vi "Main.vi"() -> ()   [LabVIEW 2017]
doc: "Use this template to build a simple state machine design pattern. Each state executes code and determines which state to transition to."
uses:
  controls/app_data.ctl
  controls/instruments.ctl
  Unicorn Labview Library/Control/unicorn_Param.ctl
  Unicorn Labview Library/Control/unicorn_conn.ctl
  Unicorn Labview Library/Control/unicorn_JSON.ctl
  Unicorn Labview Library/Control/unicorn_ParamInt.ctl
  Unicorn Labview Library/Control/unicorn_Telemetry.ctl
  Unicorn Labview Library/Control/unicorn_Table.ctl
  Unicorn Labview Library/Control/unicorn_ParamFloat.ctl
  controls/State.ctl
  <instrlib>/PICOTEST M352XA/Public/Controls/Function.ctl
  controls/attenuator_dB.ctl
  Unicorn Labview Library/Unicorn Library.lvlib
  <instrlib>/Siglent SDG X Series/Siglent SDG X Series.lvlib
panel:
  in  "app_data":T1={"Instruments"={"generator"="", "voltment_with_scaner"="", "voltment_without_scaner"=""}, "boc"={"conParam"={"ReadIntParam"=TRUE, "ReadDescrParam"=FALSE, "ReadFloatParam"=TRUE, "debug"=FALSE, "ReadJSON"=TRUE, "IP_address"="192.168.1.216", "N_attempts"=3, "type_con"=enum."TCP", "MB_address"=1, "VISA"="COM1", "connection ID"=refnum, "nameDevices"="", "timeout"=3000, "port"=2000, "type_version"="0F0C0001", "baud_rate"=115200, "VersionControl"=FALSE, "TCP_conn"=FALSE, "WindowSize"=700}, "Param"={"NumParam"={"NTelem"=0, "NInt"=0, "NFloat"=0, "NTable"=0}, "ParamInt"=[], "Telemetry"=[], "Table"=[], "ParamFloat"=[]}}, "boe"={"conParam"={"ReadIntParam"=TRUE, "ReadDescrParam"=FALSE, "ReadFloatParam"=TRUE, "debug"=FALSE, "ReadJSON"=TRUE, "IP_address"="192.168.1.216", "N_attempts"=3, "type_con"=enum."TCP", "MB_address"=1, "VISA"="COM1", "connection ID"=refnum, "nameDevices"="", "timeout"=3000, "port"=2000, "type_version"="0F0C0001", "baud_rate"=115200, "VersionControl"=FALSE, "TCP_conn"=FALSE, "WindowSize"=700}, "Param"={"NumParam"={"NTelem"=0, "NInt"=0, "NFloat"=0, "NTable"=0}, "ParamInt"=[], "Telemetry"=[], "Table"=[], "ParamFloat"=[]}}, "attenuator_tune_koef"=[]}
  out "voltmetr 3":bool
  in  "voltmetr_wothout_scaner":refnum<visa-resource-name>="voltmetr_without_scanner" caption="Вольтметр без сканера (перед аттенюатором)"
  in  "Exit":bool
  out "error out 2":errorcluster
  out "boe_connected":bool caption="Соединение"
  in  "Connect_boe":bool caption="Подключение"
  out "voltmetr":bool
  out "generator":bool
  in  "voltmetr_with_scaner":refnum<visa-resource-name>="USB0::0x164E::0x0DAD::TW00054344::INSTR" caption="Вольтметр со сканером"
  in  "generator":refnum<visa-resource-name>="generator" caption="Генератор"
  out "boc_connected":bool caption="Соединение"
  in  "Tab Control":T10(tab)
  in  "frequencies":dbl[](array[numeric])=[50000.0, 60000.0, 70000.0, 80000.0, 90000.0, 100000.0, 110000.0, 120000.0, 130000.0, 140000.0, 150000.0, 160000.0, 170000.0, 180000.0, 190000.0, 200000.0, 210000.0, 220000.0, 230000.0, 240000.0, 250000.0] format="%#_6p"
  in  "attenuator_setup":bool
  out "appended array":dbl[][](array[numeric]) format="%#_6p"
  out "после аттенюатора":dbl[](array[numeric])
  out "error out 7":errorcluster
  in  "icp_check":bool
  out "error out 3":errorcluster
  out "Telemetry 2":sgl[][](array[numeric])
  in  "calibration":bool
  out "error out 4":errorcluster
  out "meas":dbl[](array[numeric])
  out "boc_data":sgl[](array[numeric])
  out "koef":dbl[](array[numeric])
  out "meas 2":dbl[](array[numeric])
  out "boc_data 2":sgl[](array[numeric])
  out "koef 2":dbl[](array[numeric])
  in  "check_calibr":bool
  out "meas 3":dbl[](array[numeric])
  out "boc_data 3":sgl[](array[numeric])
  out "koef 3":dbl[](array[numeric])
  out "meas 4":dbl[](array[numeric])
  out "boc_data 4":sgl[](array[numeric])
  out "koef 4":dbl[](array[numeric])
  out "error out 5":errorcluster
  in  "meas_freq_char":bool
  in  "freq":dbl[](array[numeric])=[50000.0, 60000.0, 70000.0, 100000.0, 140000.0, 180000.0, 210000.0, 250000.0] caption="Частоты" format="%#_6p"
  out "error out 6":errorcluster
  in  "Tab Control 2":T11(tab)
  out "meas 5":dbl[][](array[numeric])
  out "boc_data 5":sgl[][](array[numeric])
  out "meas 6":dbl[][](array[numeric])
  out "boc_data 6":sgl[][](array[numeric])
  out "boc_data 10":sgl[][](array[numeric])
  out "meas 9":dbl[][](array[numeric])
  in  "voltage":dbl[](array[numeric])=[0.0001, 0.0005, 0.001, 0.005, 0.01, 0.05, 0.1, 0.14] min=0.0 max=1.0 format="%#_6p"
  in  "ampl_char_without_atten":bool
  out "error out 8":errorcluster
  in  "Tab Control 3":T11(tab)
  out "meas 7":dbl[][](array[numeric])
  out "boc_data 7":sgl[][](array[numeric])
  out "meas 8":dbl[][](array[numeric])
  out "boc_data 8":sgl[][](array[numeric])
  out "meas 10":dbl[][](array[numeric])
  out "boc_data 11":sgl[][](array[numeric])
  in  "cross_channel_links":bool
  out "boc_data 9":sgl[][](array[numeric])
  out "error out 9":errorcluster
  in  "Connect_boc":bool caption="Подключение"
  out "error out":errorcluster
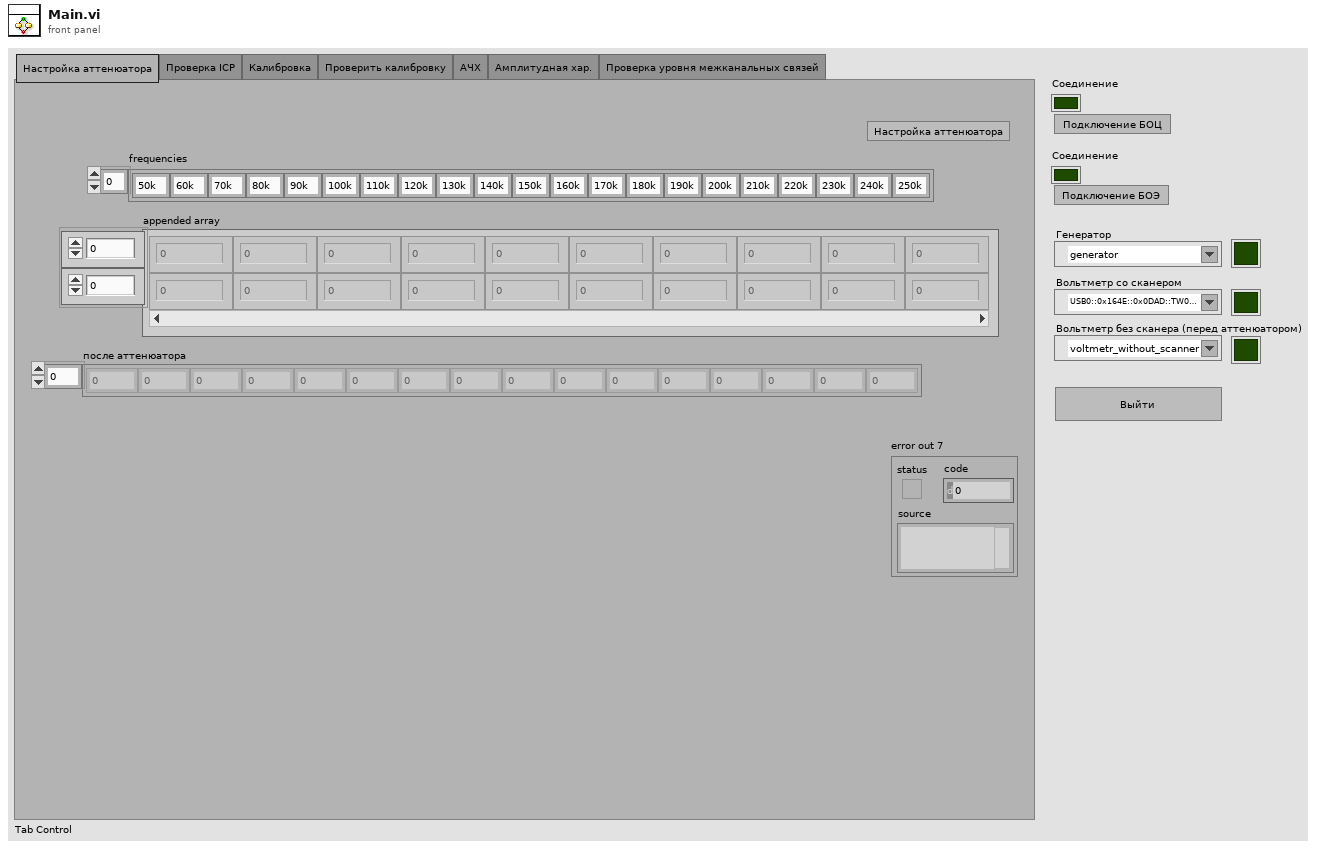
[diagram p1: front panel]
types:
  T1 = typedef "app_data.ctl" = cluster{"Instruments":T2, "boc":T3, "boe":T3, "attenuator_tune_koef":dbl[][]}
  T2 = typedef "instruments.ctl" = cluster{"generator":refnum<visa-resource-name>, "voltment_with_scaner":refnum<visa-resource-name>, "voltment_without_scaner":refnum<visa-resource-name>}
  T3 = typedef "Unicorn Library.lvlib/unicorn_Param.ctl" = cluster{"conParam":T4, "Param":T5}
  T4 = typedef "Unicorn Library.lvlib/unicorn_conn.ctl" = cluster{"ReadIntParam":bool, "ReadDescrParam":bool, "ReadFloatParam":bool, "debug":bool, "ReadJSON":bool, "IP_address":string, "N_attempts":i32, "type_con":enum16{"Serial", "TCP"}, "MB_address":i32, "VISA":refnum<visa-resource-name>, "connection ID":refnum<k5>, "nameDevices":string, "timeout":i32, "port":u16, "type_version":string, "baud_rate":u32, "VersionControl":bool, "TCP_conn":bool, "WindowSize":i32}
  T5 = typedef "Unicorn Library.lvlib/unicorn_JSON.ctl" = cluster{"NumParam":cluster{"NTelem":i32, "NInt":i32, "NFloat":i32, "NTable":i32}, "ParamInt":T6, "Telemetry":T7, "Table":T8, "ParamFloat":T9}
  T6 = typedef "Unicorn Library.lvlib/unicorn_ParamInt.ctl" = cluster{"ID":string, "Num":i32, "Name":string, "Type":string, "Enum":string, "Desc":string, "Unit":string, "Access":string, "FormatStr":string, "Min":i32, "Max":i32}[]
  T7 = typedef "Unicorn Library.lvlib/unicorn_Telemetry.ctl" = cluster{"ID":string, "Num":i32, "Name":string, "Desc":string, "Unit":string, "FormatStr":string, "Min":i32, "Max":i32}[]
  T8 = typedef "Unicorn Library.lvlib/unicorn_Table.ctl" = cluster{"Num":i32, "Access":string, "ColumnCount":i32, "NeedParamPrepare":bool, "Columns":cluster{"Column":i32, "Desc":string, "Name":string}[], "DataType":string, "FormatStr":string, "ID":string, "Name":string, "RowCount":i32, "Rows":cluster{"Desc":string, "ID":string, "Max":i32, "Min":i32, "Name":string, "Row":i32, "Unit":string}[], "Type":string}[]
  T9 = typedef "Unicorn Library.lvlib/unicorn_ParamFloat.ctl" = cluster{"ID":string, "Num":i32, "Name":string, "Type":string, "Enum":string, "Desc":string, "Unit":string, "Access":string, "FormatStr":string, "Min":i32, "Max":i32}[]
  T10 = enum32{"Настройка аттенюатора", "Проверка ICP", "Калибровка", "Проверить калибровку", "АЧХ", "Амплитудная хар.", "Проверка уровня межканальных связей"}
  T11 = enum32{"BOE -1, BOC 0", "BOE -1, BOC 3", "BOE 0, BOC 0"}
  T12 = typedef "State.ctl" = enum16{"Initialize", "Wait for Event", "User State 1", "User State 2", "Exit"}
  T13 = typedef "Function.ctl" = enum16{"VOLTage:DC", "VOLTage:DC:RATio", "VOLTage:AC", "CURRent:DC", "CURRent:AC", "RESistance", "FRESistance", "FREQuency", "PERiod", "FREQuency:CURRent", "PERiod:CURRent", "CAPacitance", "CONTinuity", "DIODe", "TCOuple", "TEMPerature"}
  T14 = typedef "attenuator_dB.ctl" = enum16{"0", "20", "40", "60"}
  T15 = typedef "Unicorn Library.lvlib/AnswerUDP.ctl" = cluster{"IP":string, "Port":u16, "DataVersion":u16, "ModbusAddress":i32, "type_version":string, "Description":string, "Serial":string, "ServerPort":u16}
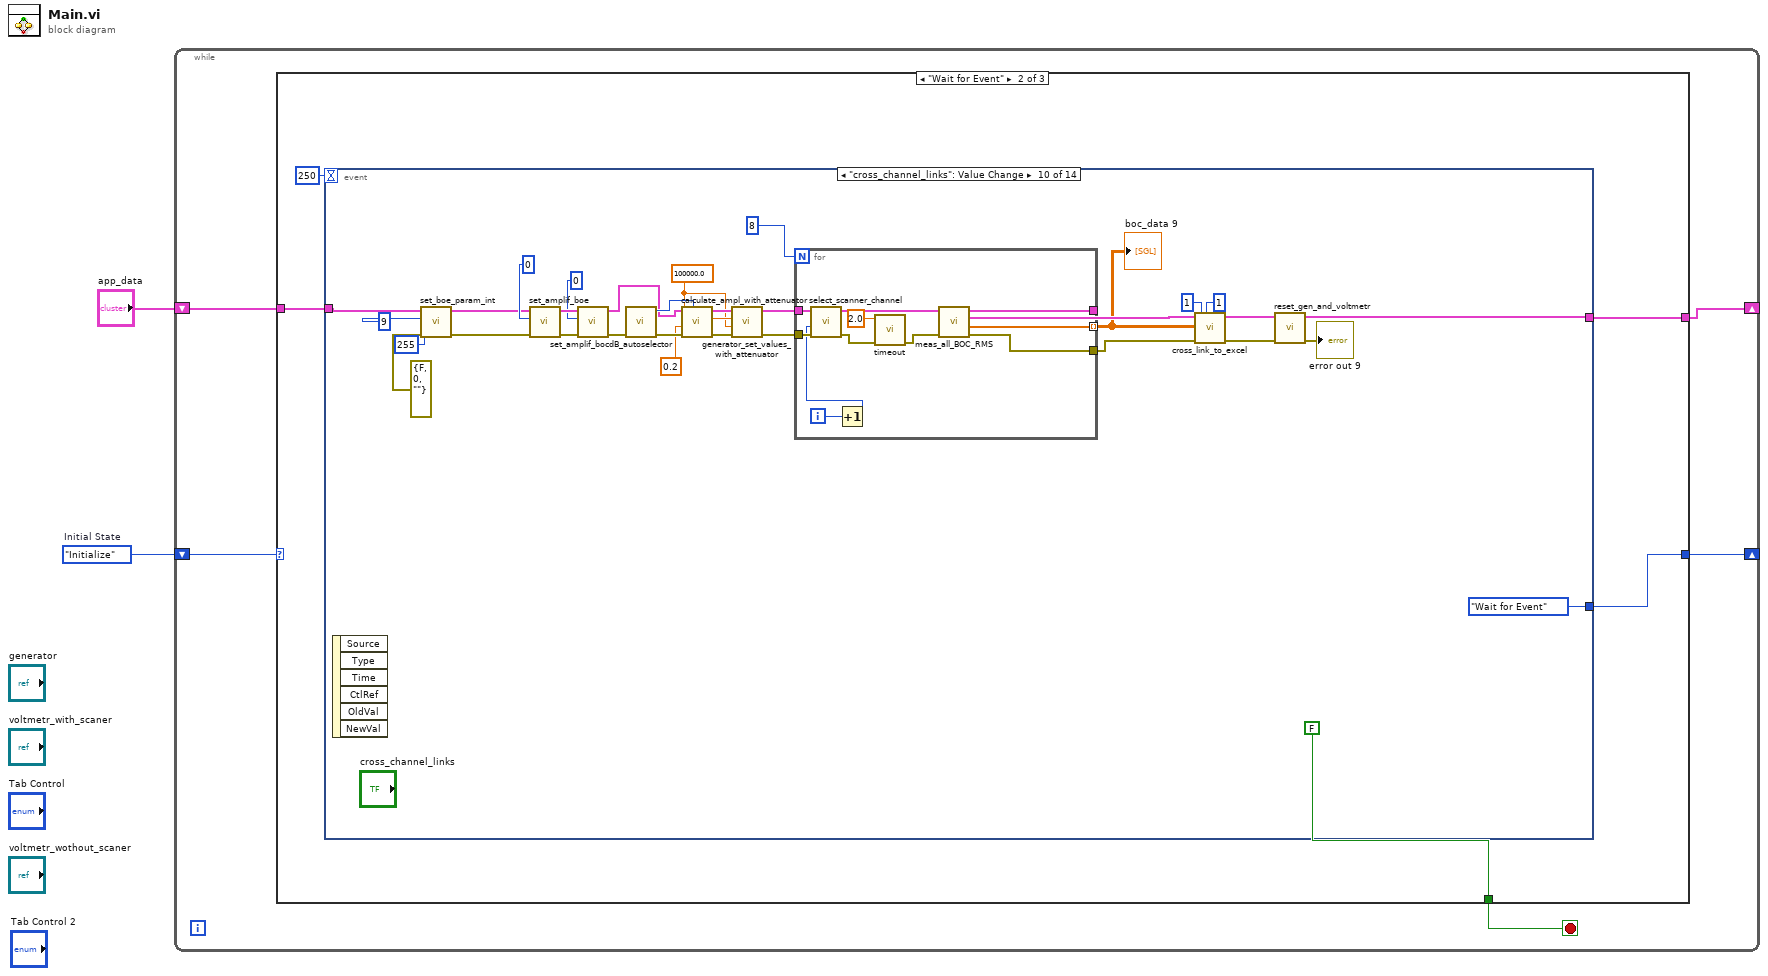
[diagram p0: block diagram]
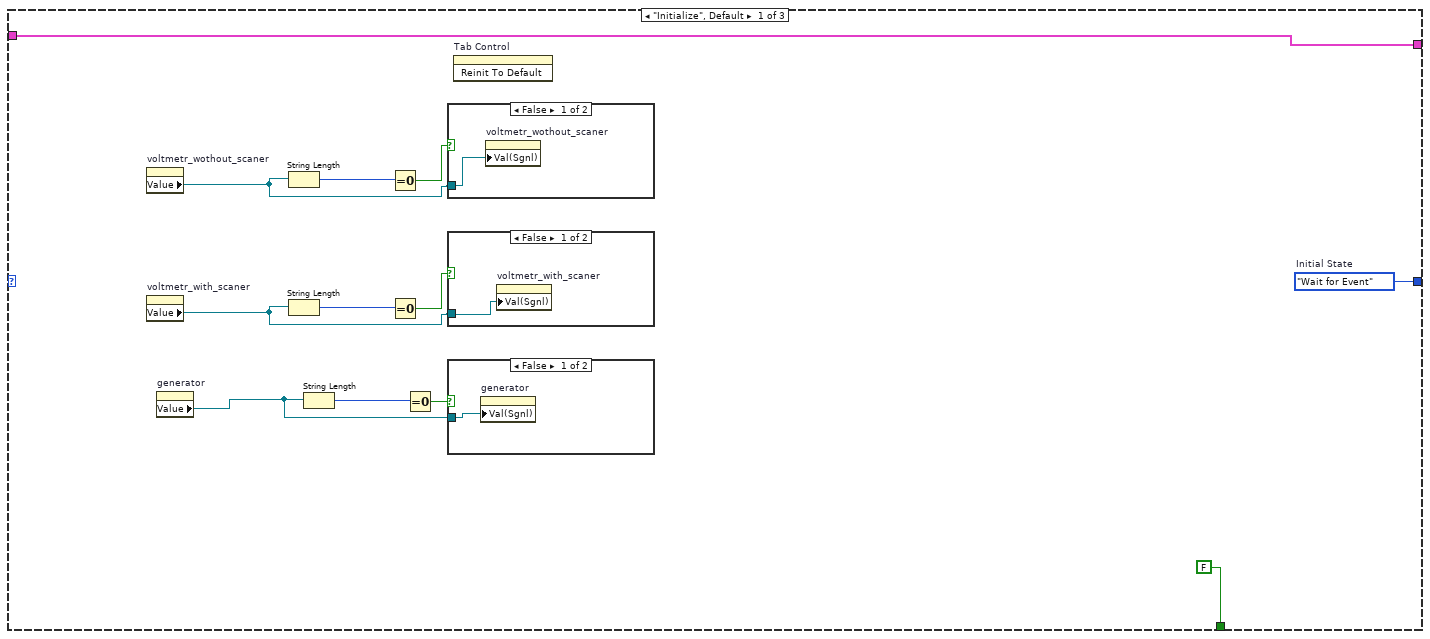
[diagram p2: hidden frame]
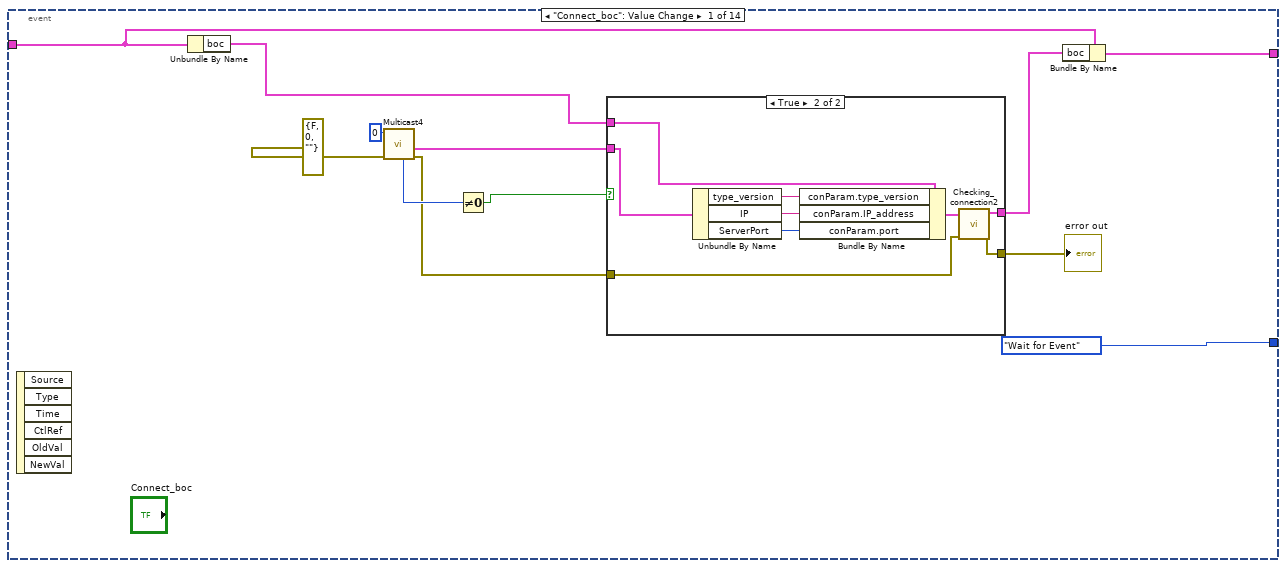
[diagram p6: hidden frame]
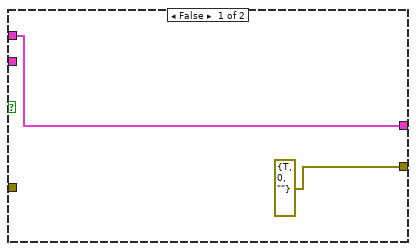
[diagram p7: hidden frame]
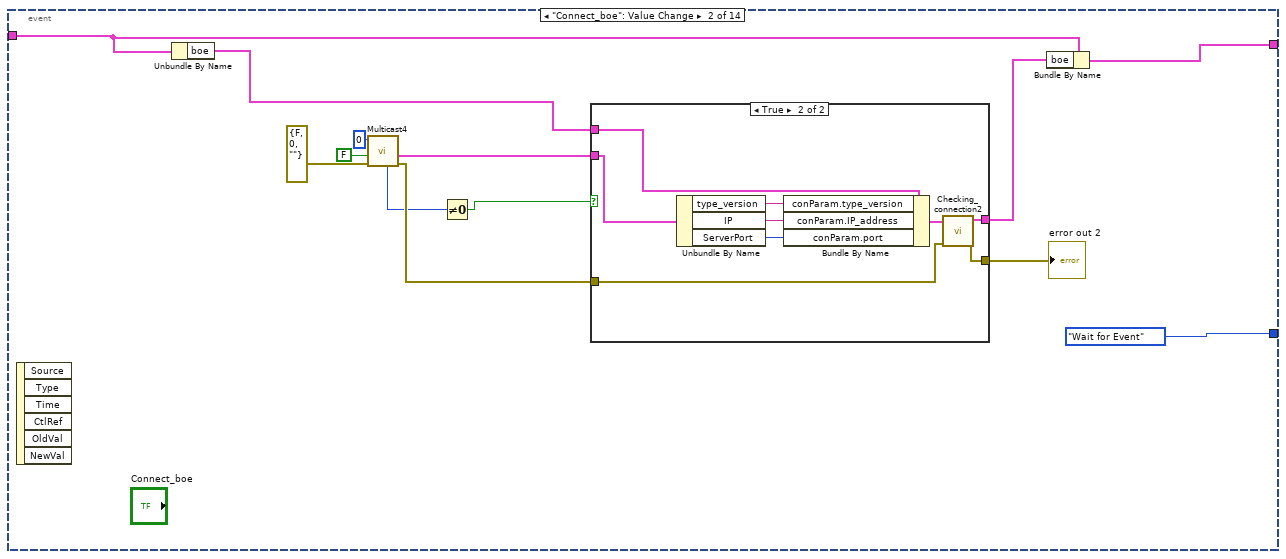
[diagram p8: hidden frame]
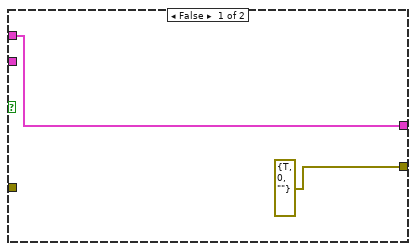
[diagram p9: hidden frame]
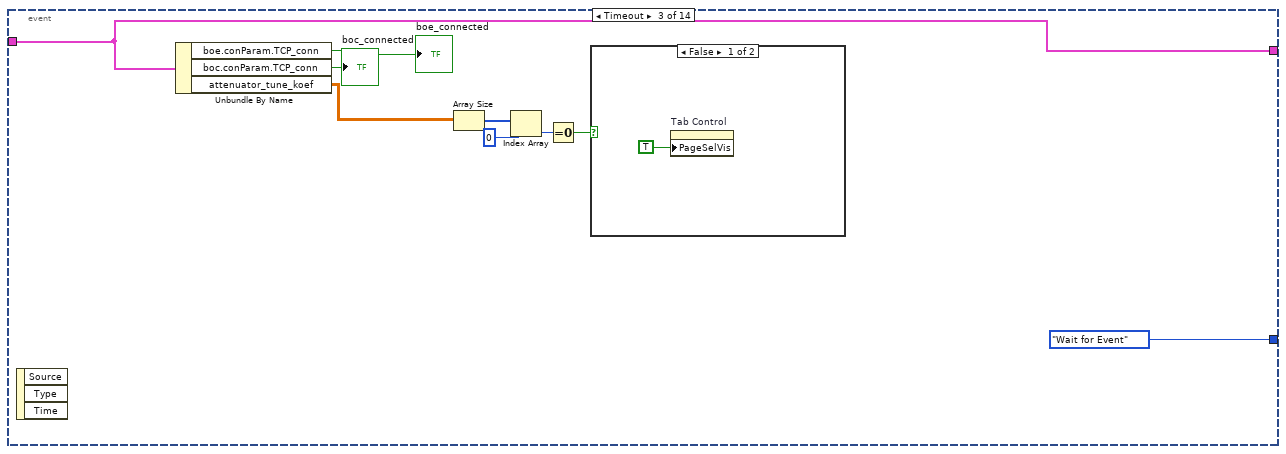
[diagram p10: hidden frame]
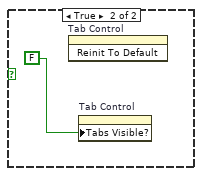
[diagram p11: hidden frame]
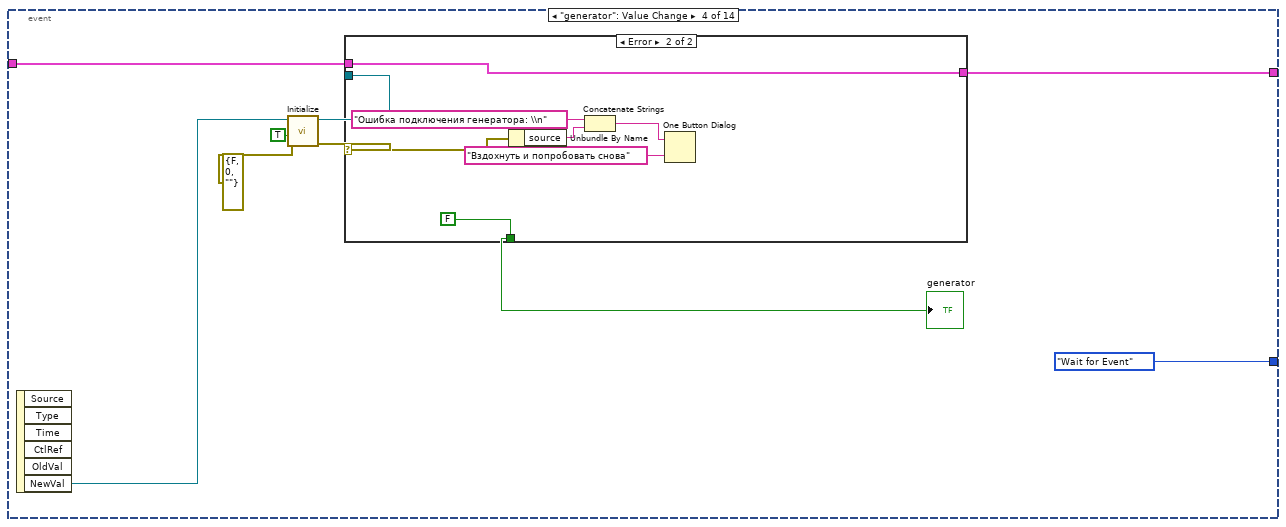
[diagram p12: hidden frame]
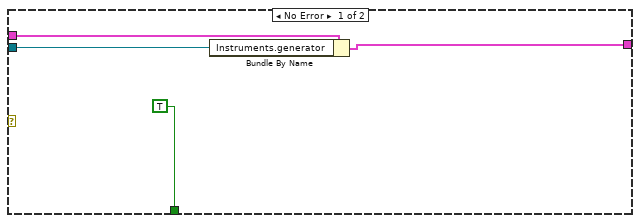
[diagram p13: hidden frame]
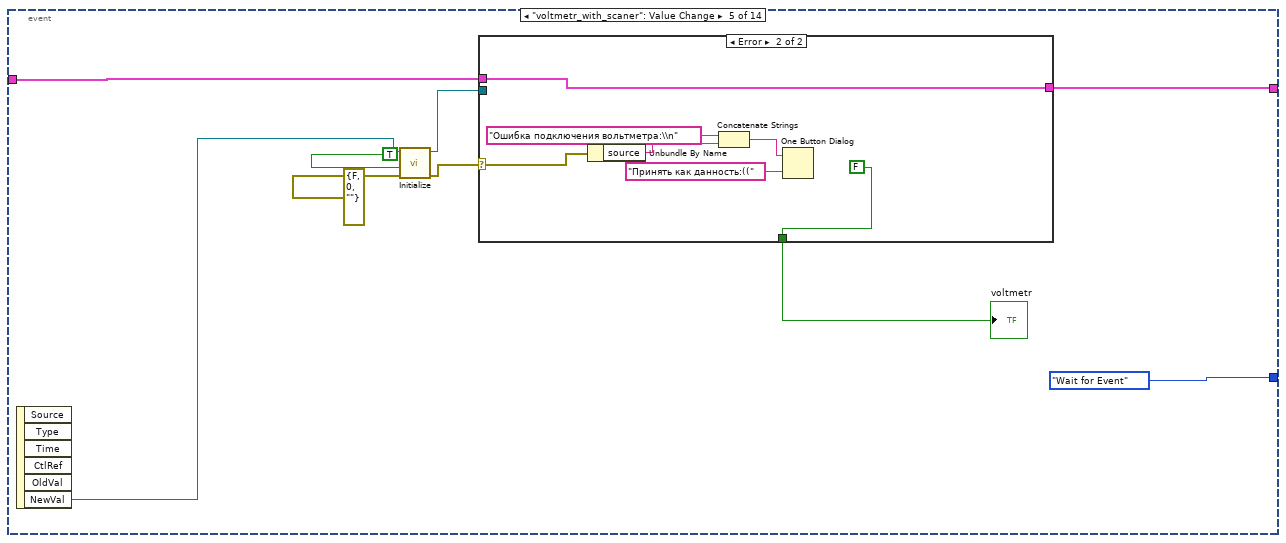
[diagram p14: hidden frame]
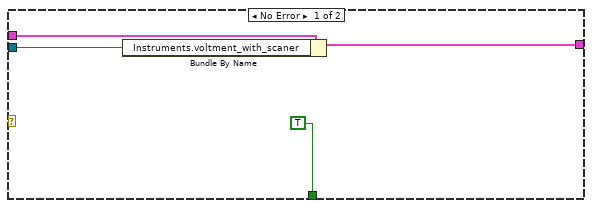
[diagram p15: hidden frame]
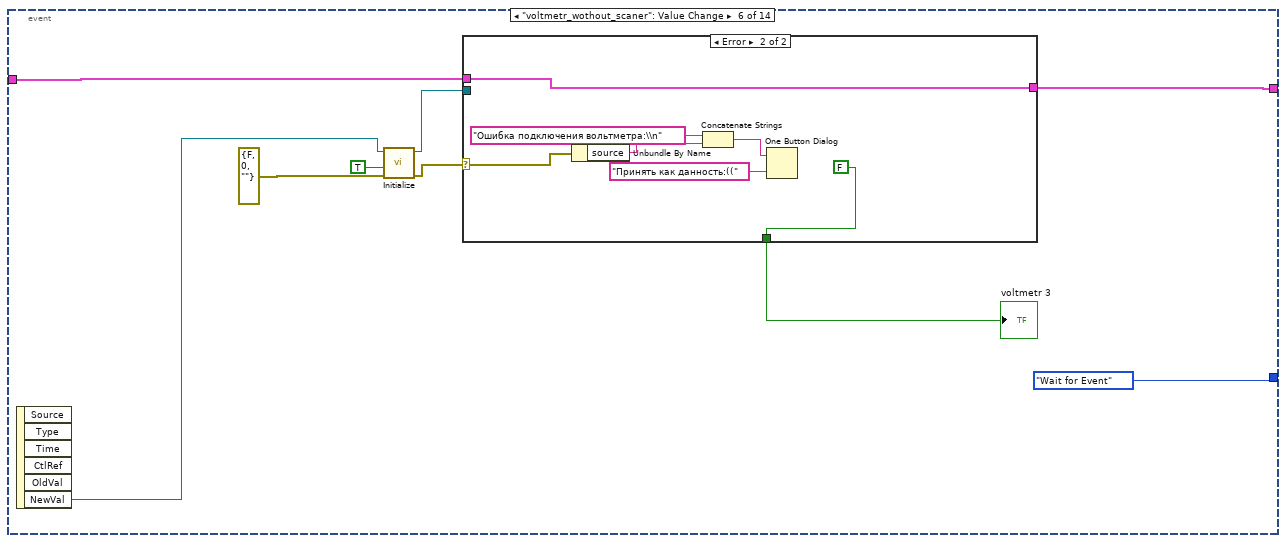
[diagram p16: hidden frame]
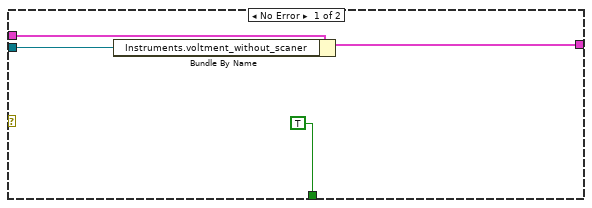
[diagram p17: hidden frame]
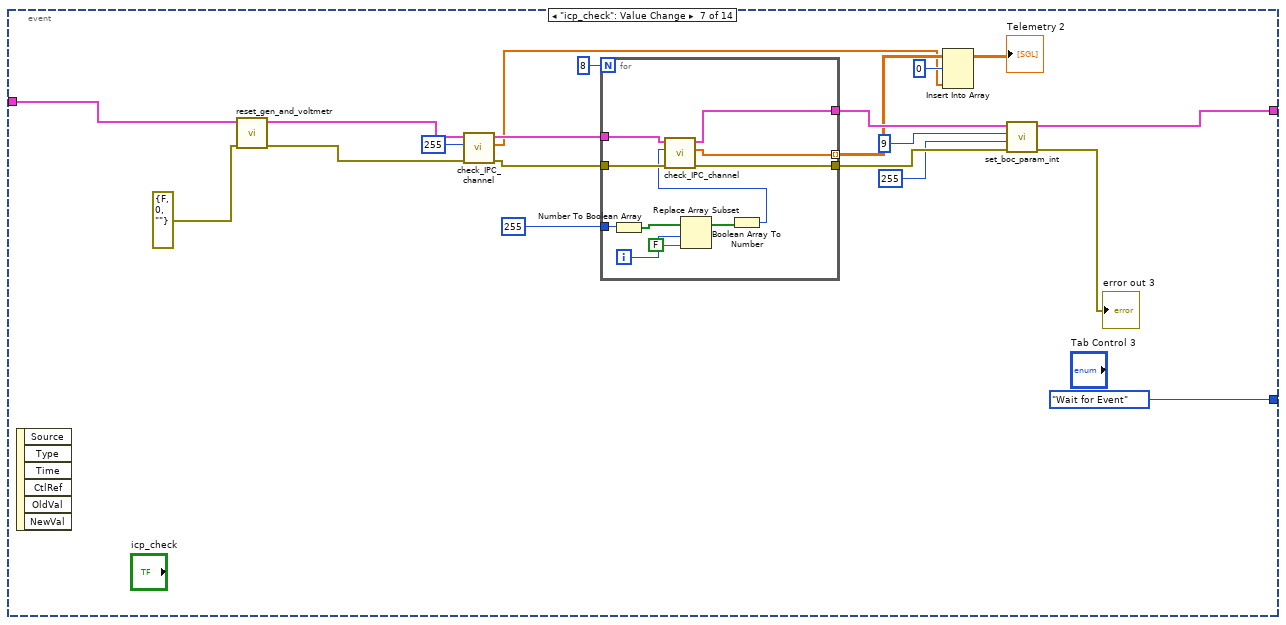
[diagram p18: hidden frame]
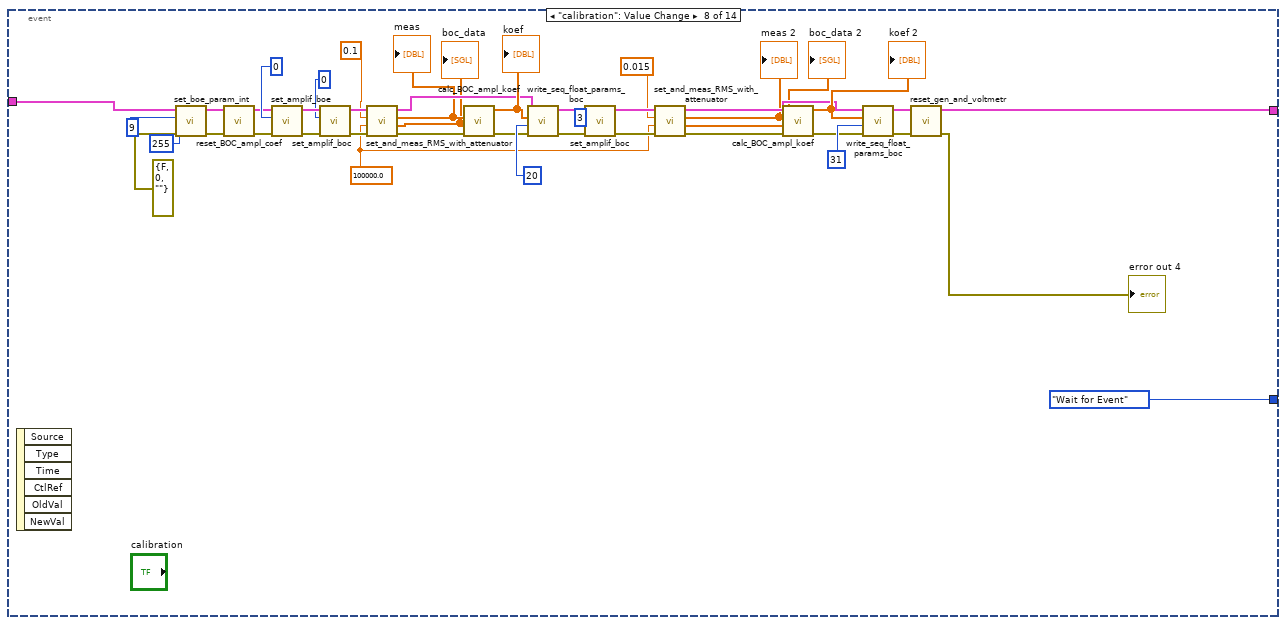
[diagram p19: hidden frame]
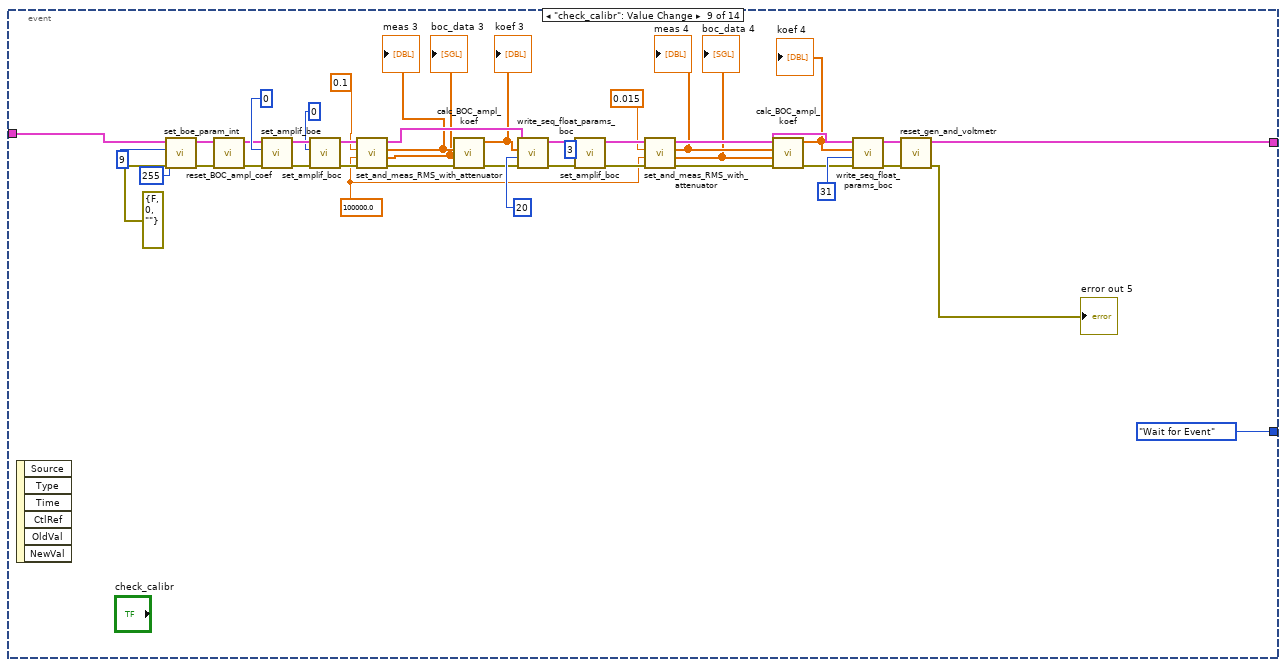
[diagram p20: hidden frame]
diagram:
  w2 = State."Initialize"  # Initial State
  n1 = while {
    shift-right: [w3] -> _
    shift-left: w2 -> [w7]
    shift-right: [w4] -> _
    shift-left: "app_data" -> [w6]
    stop <- w5 stop-if-true
    n2 = case shown="\"Wait for Event\"" w7 {
      tunnel: [w17 w25 w473] -> w4
      tunnel: w6 -> [w17 w26 w473]
      tunnel: [w19 w24 w472] -> w3
      tunnel: [FALSE FALSE TRUE] -> w5
      frame "Initialize", Default {
        w19 = State."Wait for Event"  # Initial State
        n3 = property on="voltmetr_wothout_scaner" class="VISAName"() -> ("Value"=w8:refnum<visa-resource-name>)  [unwired: 2 in, 2 out]
        n4 = property on="voltmetr_with_scaner" class="VISAName"() -> ("Value"=w11:refnum<visa-resource-name>)  [unwired: 2 in, 2 out]
        n5 = property on="generator" class="VISAName"() -> ("Value"=w14:refnum<visa-resource-name>)  [unwired: 2 in, 2 out]
        n6 = String Length(string=w8) -> (length=w9:i32)
        n7 = String Length(string=w11) -> (length=w13:i32)
        n8 = String Length(string=w14) -> (length=w16:i32)
        n9 = Equal To 0?(x=w9) -> (x = 0?=w10:bool)
        n10 = Equal To 0?(x=w13) -> (x = 0?=w12:bool)
        n11 = Equal To 0?(x=w16) -> (x = 0?=w15:bool)
        n12 = case shown="False" w10 {
          tunnel: w8 -> [w20 _]
          frame False {
            n13 = property on="voltmetr_wothout_scaner" class="VISAName"("Val(Sgnl)"=w20) -> ()  [unwired: 2 in, 2 out]
          }
          frame True {
          }
        }
        n14 = case shown="False" w12 {
          tunnel: w11 -> [w21 _]
          frame False {
            n15 = property on="voltmetr_with_scaner" class="VISAName"("Val(Sgnl)"=w21) -> ()  [unwired: 2 in, 2 out]
          }
          frame True {
          }
        }
        n16 = case shown="False" w15 {
          tunnel: w14 -> [w22 _]
          frame False {
            n17 = property on="generator" class="VISAName"("Val(Sgnl)"=w22) -> ()  [unwired: 2 in, 2 out]
          }
          frame True {
          }
        }
        n18 = invoke on="Tab Control" class="TabCtl (strict)" method="Reinit To Default"() -> ()  [unwired: 3 in, 3 out]
      }
      frame "Wait for Event" {
        n19 = event shown="[9] \"cross_channel_links\": Value Change" {
          selector: _ -> [_ _ _ _ _ _ _ _ _ _ _ _ _ _]
          dyn-events: _ -> [_ _ _ _ _ _ _ _ _ _ _ _ _ _]
          timeout: 250 -> [_ _ _ _ _ _ _ _ _ _ _ _ _ _]
          tunnel: w26 -> [w38 w53 w82 w91 w114 w130 w162 w217 w224 w283 w323 w384 w407 w464]
          tunnel: [w39 w54 w82 w89 w113 w129 w153 w194 w225 w268 w316 w383 w408 w464] -> w25
          tunnel: [State."Wait for Event" ("Initial State") State."Wait for Event" ("Initial State") State."Wait for Event" ("Initial State") State."Wait for Event" ("Initial State") State."Wait for Event" ("Initial State") State."Wait for Event" ("Initial State") State."Wait for Event" ("Initial State") State."Wait for Event" ("Initial State") State."Wait for Event" ("Initial State") State."Wait for Event" ("Initial State") State."Wait for Event" ("Initial State") State."Wait for Event" ("Initial State") State."Wait for Event" ("Initial State") State."Exit" ("Initial State")] -> w24
          event "Connect_boc": Value Change {
            n20 = event-data() -> ()  [unwired: 1 in, 6 out]
            n21 = Unbundle By Name(w38) -> ("boc"=w31:T3)
            n22 = call "Multicast4.vi"("error in"=errorcluster {"status"=FALSE, "code"=0, "source"=""} ("error in (no error)"), "type_version"=u32 0) -> ("error out"=w29:errorcluster, "selDevice"=w32:T15, "selIPhex"=w35:u32)  [unwired: 4 in, 3 out]
            n23 = Not Equal To 0?(x=w35) -> (x != 0?=w34:bool)
            n24 = case shown="True" w34 {
              tunnel: [errorcluster {"status"=TRUE, "code"=0, "source"=""} ("error out") w45] -> w33
              tunnel: w32 -> [_ w47]
              tunnel: w31 -> [w40 w46]
              tunnel: [w40 w43] -> w30
              tunnel: w29 -> [_ w42]
              frame False {
              }
              frame True {
                n25 = Unbundle By Name(w47) -> ("type_version"=w49:string, "IP"=w50:string, "ServerPort"=w48:u16)
                n26 = Bundle By Name(cluster=w46, "conParam.type_version"=w49, "conParam.IP_address"=w50, "conParam.port"=w48) -> (w44:T3)
                n27 = call "Checking_connection2.vi"("error in"=w42, "paramUnicornIn"=w44) -> ("error out"=w45:errorcluster, "paramUnicorn"=w43:T3)  [unwired: 6 in, 2 out]
              }
            }
            "error out" <- w33
            n28 = Bundle By Name(cluster=w38, "boc"=w30) -> (w39:T1)
          }
          event "Connect_boe": Value Change {
            n29 = event-data() -> ()  [unwired: 1 in, 6 out]
            n30 = Unbundle By Name(w53) -> ("boe"=w61:T3)
            n31 = call "Multicast4.vi"("error in"=errorcluster {"status"=FALSE, "code"=0, "source"=""} ("error in (no error)"), "VersionControl"=FALSE, "type_version"=u32 0) -> ("error out"=w63:errorcluster, "selDevice"=w60:T15, "selIPhex"=w57:u32)  [unwired: 3 in, 3 out]
            n32 = Not Equal To 0?(x=w57) -> (x != 0?=w58:bool)
            n33 = case shown="True" w58 {
              tunnel: [errorcluster {"status"=TRUE, "code"=0, "source"=""} ("error out") w69] -> w59
              tunnel: w60 -> [_ w71]
              tunnel: w61 -> [w64 w70]
              tunnel: [w64 w67] -> w62
              tunnel: w63 -> [_ w66]
              frame False {
              }
              frame True {
                n34 = Unbundle By Name(w71) -> ("type_version"=w73:string, "IP"=w74:string, "ServerPort"=w72:u16)
                n35 = Bundle By Name(cluster=w70, "conParam.type_version"=w73, "conParam.IP_address"=w74, "conParam.port"=w72) -> (w68:T3)
                n36 = call "Checking_connection2.vi"("error in"=w66, "paramUnicornIn"=w68) -> ("error out"=w69:errorcluster, "paramUnicorn"=w67:T3)  [unwired: 6 in, 2 out]
              }
            }
            "error out 2" <- w59
            n37 = Bundle By Name(cluster=w53, "boe"=w62) -> (w54:T1)
          }
          event Timeout {
            n38 = event-data() -> ()  [unwired: 1 in, 3 out]
            n39 = Unbundle By Name(w82) -> ("boe.conParam.TCP_conn"=→"boe_connected":bool, "boc.conParam.TCP_conn"=→"boc_connected":bool, "attenuator_tune_koef"=w79:dbl[][])
            n40 = Array Size(array=w79) -> (size(s)=w78:i32[])
            n41 = Index Array(array=w78, index=0) -> (element=w76:i32)
            n42 = Equal To 0?(x=w76) -> (x = 0?=w75:bool)
            n43 = case shown="False" w75 {
              frame False {
                n44 = property on="Tab Control" class="TabCtl (strict)"("PageSelVis"=TRUE ("Page Selector Visible")) -> ()  [unwired: 2 in, 2 out]
              }
              frame True {
                n45 = invoke on="Tab Control" class="TabCtl (strict)" method="Reinit To Default"() -> ()  [unwired: 3 in, 3 out]
                n46 = property on="Tab Control" class="TabCtl (strict)"("Tabs Visible?"=FALSE ("Page Selector Visible")) -> ()  [unwired: 2 in, 2 out]
              }
            }
          }
          event "generator": Value Change {
            n47 = event-data() -> ("NewVal"=w88:refnum<visa-resource-name>)  [unwired: 1 in, 5 out]
            n48 = call <instrlib>:"Initialize.vi"("error in (no error)"=errorcluster {"status"=FALSE, "code"=0, "source"=""}, "Reset (True)"=TRUE, "VISA resource name"=w88) -> ("error out"=w92:errorcluster, "VISA resource name out"=w90:refnum<visa-resource-name>)  [unwired: 7 in]
            n49 = case shown="Error" w92 {
              selector: w92 -> [_ w104]
              tunnel: w91 -> [w98 w105]
              tunnel: w90 -> [w97 _]
              tunnel: [w96 w105] -> w89
              tunnel: [TRUE ("generator") FALSE ("generator")] -> w87
              frame No Error {
                n50 = Bundle By Name(cluster=w98, "Instruments.generator"=w97) -> (w96:T1)
              }
              frame Error {
                n51 = Unbundle By Name(w104) -> ("source"=w103:string)
                n52 = Concatenate Strings("Ошибка подключения генератора: \\n" ("string"), w103) -> (w102:string)
                n53 = One Button Dialog(message=w102, button name ("OK")="Вздохнуть и попробовать снова") -> ()  [unwired: 1 out]
              }
            }
            "generator" <- w87
          }
          event "voltmetr_with_scaner": Value Change {
            n54 = event-data() -> ("NewVal"=w108:refnum<visa-resource-name>)  [unwired: 1 in, 5 out]
            n55 = call <instrlib>:"Initialize.vi"("error in (no error)"=errorcluster {"status"=FALSE, "code"=0, "source"=""}, "Reset (True)"=TRUE, "VISA resource name"=w108) -> ("error out"=w110:errorcluster, "VISA resource name out"=w109:refnum<visa-resource-name>)  [unwired: 6 in, 1 out]
            n56 = case shown="Error" w110 {
              selector: w110 -> [_ w124]
              tunnel: w114 -> [w118 w125]
              tunnel: [w117 w125] -> w113
              tunnel: w109 -> [w116 _]
              tunnel: [TRUE ("voltmetr") FALSE ("voltmetr")] -> w107
              frame No Error {
                n57 = Bundle By Name(cluster=w118, "Instruments.voltment_with_scaner"=w116) -> (w117:T1)
              }
              frame Error {
                n58 = Unbundle By Name(w124) -> ("source"=w123:string)
                n59 = Concatenate Strings("Ошибка подключения вольтметра:\\n" ("string"), w123) -> (w121:string)
                n60 = One Button Dialog(message=w121, button name ("OK")="Принять как данность:((") -> ()  [unwired: 1 out]
              }
            }
            "voltmetr" <- w107
          }
          event "voltmetr_wothout_scaner": Value Change {
            n61 = event-data() -> ("NewVal"=w127:refnum<visa-resource-name>)  [unwired: 1 in, 5 out]
            n62 = call <instrlib>:"Initialize.vi"("error in (no error)"=errorcluster {"status"=FALSE, "code"=0, "source"=""}, "Reset (True)"=TRUE, "VISA resource name"=w127) -> ("error out"=w132:errorcluster, "VISA resource name out"=w131:refnum<visa-resource-name>)  [unwired: 6 in, 1 out]
            n63 = case shown="Error" w132 {
              selector: w132 -> [_ w144]
              tunnel: w130 -> [w138 w145]
              tunnel: [w137 w145] -> w129
              tunnel: w131 -> [w136 _]
              tunnel: [TRUE ("voltmetr") FALSE ("voltmetr")] -> w126
              frame No Error {
                n64 = Bundle By Name(cluster=w138, "Instruments.voltment_without_scaner"=w136) -> (w137:T1)
              }
              frame Error {
                n65 = Unbundle By Name(w144) -> ("source"=w143:string)
                n66 = Concatenate Strings("Ошибка подключения вольтметра:\\n" ("string"), w143) -> (w141:string)
                n67 = One Button Dialog(message=w141, button name ("OK")="Принять как данность:((") -> ()  [unwired: 1 out]
              }
            }
            "voltmetr 3" <- w126
          }
          event "icp_check": Value Change {
            n68 = event-data() -> ()  [unwired: 1 in, 6 out]
            n69 = call "reset_gen_and_voltmetr.vi"("error in (no error)"=errorcluster {"status"=FALSE, "code"=0, "source"=""}, "app_data"=w162) -> ("error out"=w163:errorcluster, "output cluster"=w150:T1)  [unwired: 8 in]
            n70 = call "check_IPC_channel.vi"("error in (no error)"=w163, "ParamIn"=255, "app_data in"=w150) -> ("error out"=w160:errorcluster, "Telemetry"=w147:sgl[], "app_data out"=w161:T1)  [unwired: 6 in]
            n71 = for {
              N: 8 -> [_]
              tunnel: [w176] -> w149 mode=indexing
              tunnel: w161 -> [w175]
              tunnel: [w174] -> w154
              tunnel: w160 -> [w173]
              tunnel: [w172] -> w156
              tunnel: u8 255 ("ParamIn") -> [w171]
              i -> [w169]
              n72 = Number To Boolean Array(number=w171) -> (Boolean array=w170:bool[])
              n73 = Replace Array Subset(array=w170, new element=FALSE ("new element/subarray"), index=w169) -> (w167:bool[])
              n74 = Boolean Array To Number(Boolean array=w167) -> (number=w166:u32)
              n75 = call "check_IPC_channel.vi"("error in (no error)"=w173, "ParamIn"=w166, "app_data in"=w175) -> ("error out"=w172:errorcluster, "Telemetry"=w176:sgl[], "app_data out"=w174:T1)  [unwired: 6 in]
            }
            n76 = Insert Into Array(array=w149, index (row)=0, new element=w147) -> (→"Telemetry 2":sgl[][])  [unwired: 1 in]
            n77 = call "set_boс_param_int.vi"("error in (no error)"=w156, "ParamIn"=255, "NumParamIn"=9, "app_data in"=w154) -> ("error out"=→"error out 3":errorcluster, "app_data out"=w153:T1)  [unwired: 6 in]
          }
          event "calibration": Value Change {
            w182 = 100000.0 ("Frequency (1000 Hz)")
            n78 = event-data() -> ()  [unwired: 1 in, 6 out]
            n79 = call "set_boe_param_int.vi"("error in (no error)"=errorcluster {"status"=FALSE, "code"=0, "source"=""}, "ParamIn"=255, "NumParamIn"=9, "app_data in"=w217) -> ("error out"=w205:errorcluster, "app_data out"=w206:T1)  [unwired: 6 in]
            n80 = call "reset_BOC_ampl_coef.vi"("error in (no error)"=w205, "app_data in"=w206) -> ("error out"=w207:errorcluster, "app_data_out"=w208:T1)  [unwired: 8 in]
            n81 = call "set_amplif_boe.vi"("error in (no error)"=w207, "ParamIn"=0, "app_data in"=w208) -> ("error out"=w210:errorcluster, "app_data out"=w212:T1)  [unwired: 7 in]
            n82 = call "set_amplif_boc.vi"("error in (no error)"=w210, "ParamIn"=0, "app_data in"=w212) -> ("error out"=w190:errorcluster, "app_data out"=w191:T1)  [unwired: 7 in]
            n83 = call "set_and_meas_RMS_with_attenuator.vi"("error in (no error)"=w190, "Frequency (Hz)"=w182, "Amplitude (1.0 Vpp)"=0.1, "app_data in"=w191) -> ("error out"=w185:errorcluster, "boc_data"=w186:sgl[], "meas"=w187:dbl[], "output cluster out"=w188:T1)  [unwired: 4 in]
            "meas" <- w187
            "boc_data" <- w186
            n84 = call "calc_BOC_ampl_koef.vi"("error_in"=w185, "boc_data"=w186, "meas"=w187) -> ("error_out"=w192:errorcluster, "koef"=w204:dbl[])  [unwired: 7 in]
            "koef" <- w204
            n85 = call "write_seq_float_params_boc.vi"("error in"=w192, "Стартовый номер параметра"=20, "data"=w204, "app_data_in"=w188) -> ("error out"=w202:errorcluster, "app_data_out"=w201:T1)  [unwired: 6 in]
            n86 = call "set_amplif_boc.vi"("error in (no error)"=w202, "ParamIn"=3, "app_data in"=w201) -> ("error out"=w183:errorcluster, "app_data out"=w184:T1)  [unwired: 7 in]
            n87 = call "set_and_meas_RMS_with_attenuator.vi"("error in (no error)"=w183, "Frequency (Hz)"=w182, "Amplitude (1.0 Vpp)"=0.015, "app_data in"=w184) -> ("error out"=w180:errorcluster, "boc_data"=w178:sgl[], "meas"=w179:dbl[], "output cluster out"=w181:T1)  [unwired: 4 in]
            "meas 2" <- w179
            "boc_data 2" <- w178
            n88 = call "calc_BOC_ampl_koef.vi"("error_in"=w180, "boc_data"=w178, "meas"=w179) -> ("error_out"=w197:errorcluster, "koef"=w199:dbl[])  [unwired: 7 in]
            "koef 2" <- w199
            n89 = call "write_seq_float_params_boc.vi"("error in"=w197, "Стартовый номер параметра"=31, "data"=w199, "app_data_in"=w181) -> ("error out"=w196:errorcluster, "app_data_out"=w195:T1)  [unwired: 6 in]
            n90 = call "reset_gen_and_voltmetr.vi"("error in (no error)"=w196, "app_data"=w195) -> ("error out"=→"error out 4":errorcluster, "output cluster"=w194:T1)  [unwired: 8 in]
          }
          event "check_calibr": Value Change {
            w229 = 100000.0 ("Frequency (1000 Hz)")
            n91 = event-data() -> ()  [unwired: 1 in, 6 out]
            n92 = call "set_boe_param_int.vi"("error in (no error)"=errorcluster {"status"=FALSE, "code"=0, "source"=""}, "ParamIn"=255, "NumParamIn"=9, "app_data in"=w224) -> ("error out"=w247:errorcluster, "app_data out"=w248:T1)  [unwired: 6 in]
            n93 = call "reset_BOC_ampl_coef.vi"("error in (no error)"=w247, "app_data in"=w248) -> ("error out"=w249:errorcluster, "app_data_out"=w250:T1)  [unwired: 8 in]
            n94 = call "set_amplif_boe.vi"("error in (no error)"=w249, "ParamIn"=0, "app_data in"=w250) -> ("error out"=w252:errorcluster, "app_data out"=w254:T1)  [unwired: 7 in]
            n95 = call "set_amplif_boc.vi"("error in (no error)"=w252, "ParamIn"=0, "app_data in"=w254) -> ("error out"=w235:errorcluster, "app_data out"=w236:T1)  [unwired: 7 in]
            n96 = call "set_and_meas_RMS_with_attenuator.vi"("error in (no error)"=w235, "Frequency (Hz)"=w229, "Amplitude (1.0 Vpp)"=0.1, "app_data in"=w236) -> ("error out"=w232:errorcluster, "boc_data"=w222:sgl[], "meas"=w223:dbl[], "output cluster out"=w233:T1)  [unwired: 4 in]
            "meas 3" <- w223
            "boc_data 3" <- w222
            n97 = call "calc_BOC_ampl_koef.vi"("error_in"=w232, "boc_data"=w222, "meas"=w223) -> ("error_out"=w237:errorcluster, "koef"=w221:dbl[])  [unwired: 7 in]
            "koef 3" <- w221
            n98 = call "write_seq_float_params_boc.vi"("error in"=w237, "Стартовый номер параметра"=20, "data"=w221, "app_data_in"=w233) -> ("error out"=w245:errorcluster, "app_data_out"=w244:T1)  [unwired: 6 in]
            n99 = call "set_amplif_boc.vi"("error in (no error)"=w245, "ParamIn"=3, "app_data in"=w244) -> ("error out"=w230:errorcluster, "app_data out"=w231:T1)  [unwired: 7 in]
            n100 = call "set_and_meas_RMS_with_attenuator.vi"("error in (no error)"=w230, "Frequency (Hz)"=w229, "Amplitude (1.0 Vpp)"=0.015, "app_data in"=w231) -> ("error out"=w227:errorcluster, "boc_data"=w219:sgl[], "meas"=w220:dbl[], "output cluster out"=w228:T1)  [unwired: 4 in]
            "meas 4" <- w220
            "boc_data 4" <- w219
            n101 = call "calc_BOC_ampl_koef.vi"("error_in"=w227, "boc_data"=w219, "meas"=w220) -> ("error_out"=w241:errorcluster, "koef"=w218:dbl[])  [unwired: 7 in]
            "koef 4" <- w218
            n102 = call "write_seq_float_params_boc.vi"("error in"=w241, "Стартовый номер параметра"=31, "data"=w218, "app_data_in"=w228) -> ("error out"=w240:errorcluster, "app_data_out"=w239:T1)  [unwired: 6 in]
            n103 = call "reset_gen_and_voltmetr.vi"("error in (no error)"=w240, "app_data"=w239) -> ("error out"=→"error out 5":errorcluster, "output cluster"=w225:T1)  [unwired: 8 in]
          }
          event "cross_channel_links": Value Change {
            w273 = 100000.0 ("frequency")
            n104 = event-data() -> ()  [unwired: 1 in, 6 out]
            n105 = call "set_boe_param_int.vi"("error in (no error)"=errorcluster {"status"=FALSE, "code"=0, "source"=""}, "ParamIn"=255, "NumParamIn"=9, "app_data in"=w283) -> ("error out"=w259:errorcluster, "app_data out"=w260:T1)  [unwired: 6 in]
            n106 = call "set_amplif_boe.vi"("error in (no error)"=w259, "ParamIn"=0, "app_data in"=w260) -> ("error out"=w285:errorcluster, "app_data out"=w287:T1)  [unwired: 7 in]
            n107 = call "set_amplif_boc.vi"("error in (no error)"=w285, "ParamIn"=0, "app_data in"=w287) -> ("error out"=w281:errorcluster, "app_data out"=w278:T1)  [unwired: 7 in]
            n108 = call "dB_autoselector.vi"("error_in"=w281) -> ("error_out"=w280:errorcluster, "Attenuator(dB)"=w279:T14)  [unwired: 9 in]
            n109 = call "calculate_ampl_with_attenuator.vi"("Attenuator(dB)"=w279, "error in"=w280, "Amplitude_in"=0.2, "frequency"=w273, "app_data in in"=w278) -> ("error out"=w276:errorcluster, "Amplitude_out"=w275:dbl, "app_data out"=w274:T1)  [unwired: 4 in]
            n110 = call "generator_set_values_with_attenuator.vi"("error in (no error)"=w276, "Frequency (1000 Hz)"=w273, "Amplitude (1.0 Vpp)"=w275, "app_data"=w274) -> ("error out"=w270:errorcluster, "output cluster"=w271:T1)  [unwired: 6 in]
            n111 = for {
              N: 8 -> [_]
              tunnel: w271 -> [w300]
              tunnel: w270 -> [w299]
              tunnel: [w295] -> w269
              tunnel: [w294] -> w262 mode=indexing
              tunnel: [w293] -> w264
              i -> [w297]
              n112 = Increment(x=w297) -> (x+1=w296:i32)
              n113 = call "select_scanner_channel.vi"("error in (no error)"=w299, "channel"=w296, "output cluster"=w300) -> ("error out"=w292:errorcluster, "output cluster 2"=w298:T1)  [unwired: 7 in]
              n114 = call "timeout.vi"("error in (no error)"=w292, "seconds to wait"=2.0) -> ("error IO"=w291:errorcluster)  [unwired: 9 in]
              n115 = call "meas_all_BOC_RMS.vi"("error in (no error)"=w291, "output cluster in"=w298) -> ("error out"=w293:errorcluster, "boc_data"=w294:sgl[], "output cluster out"=w295:T1)  [unwired: 7 in]
            }
            "boc_data 9" <- w262
            n116 = call "cross_link_to_excel.vi"("error in (no error)"=w264, "position (excel).row"=1, "position (excel).column"=1, "boc_data"=w262) -> ("error out"=w263:errorcluster)  [unwired: 7 in]
            n117 = call "reset_gen_and_voltmetr.vi"("error in (no error)"=w263, "app_data"=w269) -> ("error out"=→"error out 9":errorcluster, "output cluster"=w268:T1)  [unwired: 8 in]
          }
          event "attenuator_setup": Value Change {
            n118 = event-data() -> ()  [unwired: 1 in, 6 out]
            n119 = Two Button Dialog(message="Установите аттенюатор на значение 0dB") -> (T button?=w303:bool)  [unwired: 2 in]
            n120 = case shown="False" w303 {
              tunnel: [errorcluster {"status"=TRUE, "code"=1, "source"="Отменено"} ("error in (no error)") errorcluster {"status"=FALSE, "code"=0, "source"=""} ("error in (no error)")] -> w322
              frame False {
              }
              frame True {
              }
            }
            n121 = call "reset_all_devices.vi"("error in (no error)"=w322, "app_data in"=w323) -> ("error out"=w318:errorcluster, "app_data out"=w319:T1)  [unwired: 8 in]
            n122 = call "set_boe_param_int.vi"("error in (no error)"=w318, "ParamIn"=255, "NumParamIn"=9, "app_data in"=w319) -> ("error out"=w313:errorcluster, "app_data out"=w314:T1)  [unwired: 6 in]
            n123 = call "select_scanner_channel.vi"("error in (no error)"=w313, "channel"=1, "output cluster"=w314) -> ("error out"=w310:errorcluster, "output cluster 2"=w311:T1)  [unwired: 7 in]
            n124 = for {
              tunnel: [w332] -> w307
              tunnel: [w331] -> w301
              tunnel: "frequencies" -> [w342] mode=indexing
              tunnel: w311 -> [w341]
              tunnel: w310 -> [w334]
              tunnel: [w333] -> w308 mode=indexing
              tunnel: [w335] -> w302 mode=indexing
              stop <- w334 stop-if-true
              w330 = 1.0 ("Amplitude (1.0 Vpp)")
              (unwired) Function."VOLTage:AC" ("Function")
              n125 = call "generator_set_values_with_attenuator.vi"("error in (no error)"=w334, "Frequency (1000 Hz)"=w342, "Amplitude (1.0 Vpp)"=w330, "app_data"=w341) -> ("error out"=w338:errorcluster, "output cluster"=w340:T1)  [unwired: 6 in]
              n126 = call "timeout.vi"("error in (no error)"=w338, "seconds to wait"=1.0) -> ("error IO"=w337:errorcluster)  [unwired: 9 in]
              n127 = call "meas_voltmetr_with_scanner.vi"("error in (no error)"=w337, "Function"=Function."VOLTage:AC", "output cluster in"=w340) -> ("error out"=w331:errorcluster, "value"=w335:dbl, "output cluster out"=w332:T1)  [unwired: 6 in]
              n128 = Divide(x=w330, y=w335) -> (x/y=w333:dbl)
            }
            "после аттенюатора" <- w302
            n129 = case shown="No Error" w301 {
              tunnel: "frequencies" -> [w326 _]
              tunnel: w308 -> [w325 _]
              tunnel: [w324 dbl[][] []] -> w306
              frame No Error {
                n130 = Build Array(w326, w325) -> (w324:dbl[][])
              }
              frame Error {
              }
            }
            "appended array" <- w306
            n131 = Bundle By Name(cluster=w307, "attenuator_tune_koef"=w306) -> (w305:T1)
            n132 = call "reset_all_devices.vi"("error in (no error)"=w301, "app_data in"=w305) -> ("error out"=→"error out 7":errorcluster, "app_data out"=w316:T1)  [unwired: 8 in]
          }
          event "meas_freq_char": Value Change {
            n133 = event-data() -> ()  [unwired: 1 in, 6 out]
            n134 = call "set_boe_param_int.vi"("error in (no error)"=errorcluster {"status"=FALSE, "code"=0, "source"=""}, "ParamIn"=255, "NumParamIn"=9, "app_data in"=w384) -> ("error out"=w387:errorcluster, "app_data out"=w388:T1)  [unwired: 6 in]
            n135 = call "set_amplif_boe.vi"("error in (no error)"=w387, "ParamIn"=-1, "app_data in"=w388) -> ("error out"=w394:errorcluster, "app_data out"=w396:T1)  [unwired: 7 in]
            n136 = call "set_amplif_boc.vi"("error in (no error)"=w394, "ParamIn"=0, "app_data in"=w396) -> ("error out"=w393:errorcluster, "app_data out"=w392:T1)  [unwired: 7 in]
            n137 = call "check_boc_rms_freq_char.vi"("Attenuator(dB)"=attenuator_dB."40", "error in (no error)"=w393, "Amplitude (1.0 Vpp)"=0.015, "freq"="freq", "app_data in"=w392) -> ("error out"=w386:errorcluster, "meas"=w379:dbl[][], "boc_data"=w380:sgl[][], "app_data_out"=w378:T1)  [unwired: 3 in]
            "meas 5" <- w379
            "boc_data 5" <- w380
            n138 = call "set_amplif_boc.vi"("error in (no error)"=w386, "ParamIn"=3, "app_data in"=w378) -> ("error out"=w375:errorcluster, "app_data out"=w374:T1)  [unwired: 7 in]
            n139 = call "check_boc_rms_freq_char.vi"("need_attenuator_notification"=FALSE, "Attenuator(dB)"=attenuator_dB."40", "error in (no error)"=w375, "Amplitude (1.0 Vpp)"=0.015, "freq"="freq", "app_data in"=w374) -> ("error out"=w371:errorcluster, "meas"=w368:dbl[][], "boc_data"=w369:sgl[][], "app_data_out"=w370:T1)  [unwired: 2 in]
            "meas 6" <- w368
            "boc_data 6" <- w369
            n140 = call "set_amplif_boe.vi"("error in (no error)"=w371, "ParamIn"=0, "app_data in"=w370) -> ("error out"=w365:errorcluster, "app_data out"=w366:T1)  [unwired: 7 in]
            n141 = call "set_amplif_boc.vi"("error in (no error)"=w365, "ParamIn"=0, "app_data in"=w366) -> ("error out"=w362:errorcluster, "app_data out"=w363:T1)  [unwired: 7 in]
            n142 = call "check_boc_rms_freq_char.vi"("need_attenuator_notification"=FALSE, "Attenuator(dB)"=attenuator_dB."40", "error in (no error)"=w362, "Amplitude (1.0 Vpp)"=0.015, "freq"="freq", "app_data in"=w363) -> ("error out"=w350:errorcluster, "meas"=w358:dbl[][], "boc_data"=w359:sgl[][], "app_data_out"=w351:T1)  [unwired: 2 in]
            "boc_data 10" <- w359
            "meas 9" <- w358
            n143 = call "set_amplif_boc.vi"("error in (no error)"=w350, "ParamIn"=3, "app_data in"=w351) -> ("error out"=w355:errorcluster, "app_data out"=w354:T1)  [unwired: 7 in]
            n144 = call "check_boc_rms_freq_char.vi"("need_attenuator_notification"=FALSE, "Attenuator(dB)"=attenuator_dB."40", "error in (no error)"=w355, "Amplitude (1.0 Vpp)"=0.015, "freq"="freq", "app_data in"=w354) -> ("error out"=w352:errorcluster, "meas"=w347:dbl[][], "boc_data"=w348:sgl[][], "app_data_out"=w346:T1)  [unwired: 2 in]
            n145 = call "assembly_freq_result.vi"("meas_koef_0_0"=w358, "boc_data_koef_0_0"=w359, "meas_koef_0_3"=w347, "meas_koef_-1_0"=w379, "boc_data_koef_0_3"=w348, "error in (no error)"=w352, "boc_data_koef_-1_0"=w380, "meas_koef_-1_3"=w368, "boc_data_koef_-1_3"=w369) -> ("error out"=w382:errorcluster)  [unwired: 2 in]
            n146 = call "reset_gen_and_voltmetr.vi"("error in (no error)"=w382, "app_data"=w346) -> ("error out"=→"error out 6":errorcluster, "output cluster"=w383:T1)  [unwired: 8 in]
          }
          event "ampl_char_without_atten": Value Change {
            n147 = event-data() -> ()  [unwired: 1 in, 6 out]
            n148 = call "set_boe_param_int.vi"("error in (no error)"=errorcluster {"status"=FALSE, "code"=0, "source"=""}, "ParamIn"=255, "NumParamIn"=9, "app_data in"=w407) -> ("error out"=w414:errorcluster, "app_data out"=w415:T1)  [unwired: 6 in]
            n149 = for {
              tunnel: "voltage" -> [w425] mode=indexing
              tunnel: w415 -> [w456]
              tunnel: [w433] -> w411
              tunnel: w414 -> [w455]
              tunnel: [w434] -> w410
              tunnel: [w442] -> w406 mode=indexing
              tunnel: [w441] -> w405 mode=indexing
              tunnel: [w440] -> w404 mode=indexing
              tunnel: [w439] -> w403 mode=indexing
              tunnel: [w438] -> w402 mode=indexing
              tunnel: [w437] -> w401 mode=indexing
              tunnel: [w424] -> w400 mode=indexing
              tunnel: [w423] -> w399 mode=indexing
              w426 = 100000.0 ("Frequency (Hz)")
              n150 = call "set_amplif_boe.vi"("error in (no error)"=w455, "ParamIn"=-1, "app_data in"=w456) -> ("error out"=w461:errorcluster, "app_data out"=w463:T1)  [unwired: 7 in]
              n151 = call "set_amplif_boc.vi"("error in (no error)"=w461, "ParamIn"=0, "app_data in"=w463) -> ("error out"=w460:errorcluster, "app_data out"=w459:T1)  [unwired: 7 in]
              n152 = call "set_and_meas_RMS_with_attenuator.vi"("error in (no error)"=w460, "Frequency (Hz)"=w426, "Amplitude (1.0 Vpp)"=w425, "app_data in"=w459) -> ("error out"=w454:errorcluster, "boc_data"=w441:sgl[], "meas"=w442:dbl[], "output cluster out"=w453:T1)  [unwired: 4 in]
              n153 = call "set_amplif_boc.vi"("error in (no error)"=w454, "ParamIn"=3, "app_data in"=w453) -> ("error out"=w452:errorcluster, "app_data out"=w451:T1)  [unwired: 7 in]
              n154 = call "set_and_meas_RMS_with_attenuator.vi"("need_attenuator_notification"=FALSE, "error in (no error)"=w452, "Frequency (Hz)"=w426, "Amplitude (1.0 Vpp)"=w425, "app_data in"=w451) -> ("error out"=w450:errorcluster, "boc_data"=w439:sgl[], "meas"=w440:dbl[], "output cluster out"=w449:T1)  [unwired: 3 in]
              n155 = call "set_amplif_boe.vi"("error in (no error)"=w450, "ParamIn"=0, "app_data in"=w449) -> ("error out"=w446:errorcluster, "app_data out"=w447:T1)  [unwired: 7 in]
              n156 = call "set_amplif_boc.vi"("error in (no error)"=w446, "ParamIn"=0, "app_data in"=w447) -> ("error out"=w443:errorcluster, "app_data out"=w444:T1)  [unwired: 7 in]
              n157 = call "set_and_meas_RMS_with_attenuator.vi"("need_attenuator_notification"=FALSE, "error in (no error)"=w443, "Frequency (Hz)"=w426, "Amplitude (1.0 Vpp)"=w425, "app_data in"=w444) -> ("error out"=w429:errorcluster, "boc_data"=w437:sgl[], "meas"=w438:dbl[], "output cluster out"=w430:T1)  [unwired: 3 in]
              n158 = call "set_amplif_boe.vi"("error in (no error)"=w429, "ParamIn"=0, "app_data in"=w430) -> ("error out"=w431:errorcluster, "app_data out"=w432:T1)  [unwired: 7 in]
              n159 = call "set_amplif_boc.vi"("error in (no error)"=w431, "ParamIn"=3, "app_data in"=w432) -> ("error out"=w436:errorcluster, "app_data out"=w435:T1)  [unwired: 7 in]
              n160 = call "set_and_meas_RMS_with_attenuator.vi"("need_attenuator_notification"=FALSE, "error in (no error)"=w436, "Frequency (Hz)"=w426, "Amplitude (1.0 Vpp)"=w425, "app_data in"=w435) -> ("error out"=w434:errorcluster, "boc_data"=w424:sgl[], "meas"=w423:dbl[], "output cluster out"=w433:T1)  [unwired: 3 in]
            }
            "meas 7" <- w406
            "boc_data 7" <- w405
            "meas 8" <- w404
            "boc_data 8" <- w403
            "meas 10" <- w402
            "boc_data 11" <- w401
            n161 = call "assembly_amp_0dB_result.vi"("meas_koef_0_0"=w402, "boc_data_koef_0_0"=w401, "meas_koef_0_3"=w399, "meas_koef_-1_0"=w406, "boc_data_koef_0_3"=w400, "error in (no error)"=w410, "boc_data_koef_-1_0"=w405, "meas_koef_-1_3"=w404, "boc_data_koef_-1_3"=w403) -> ("error out"=w412:errorcluster)  [unwired: 2 in]
            n162 = call "reset_gen_and_voltmetr.vi"("error in (no error)"=w412, "app_data"=w411) -> ("error out"=→"error out 8":errorcluster, "output cluster"=w408:T1)  [unwired: 8 in]
          }
          event "Exit": Value Change {
            n163 = event-data() -> ()  [unwired: 1 in, 6 out]
            n164 = Unbundle By Name(w464) -> ("boc"=w466:T3, "boe"=w465:T3)
            n165 = Unbundle By Name(w466) -> ("conParam.TCP_conn"=w467:bool)
            n166 = Unbundle By Name(w465) -> ("conParam.TCP_conn"=w468:bool)
            n167 = case shown="True" w467 {
              tunnel: w466 -> [_ w471]
              frame False {
              }
              frame True {
                n168 = call "Disconnect (SubVI).vi"("paramUnicornIn"=w471) -> ()  [unwired: 9 in, 2 out]
              }
            }
            n169 = case shown="True" w468 {
              tunnel: w465 -> [_ w470]
              frame False {
              }
              frame True {
                n170 = call "Disconnect (SubVI).vi"("paramUnicornIn"=w470) -> ()  [unwired: 9 in, 2 out]
              }
            }
          }
        }
      }
      frame "Exit" {
        w472 = State."Exit"  # Initial State
      }
    }
  }
